vi "Error Check.vi"(8 "Error In":errorcluster, 9 "Next State Queue":refnum<queue>, 10 "Acquired Traces Queue":refnum<queue>) -> (0 "error out":errorcluster, 1 "Next State Queue":refnum<queue>, 2 "Acquired Traces Queue":refnum<queue>, 4 "Next State":T1, 5 "Error":bool)   [LabVIEW 2019]
uses:
  Controls/DAQ States.ctl
  Controls/Acquisition Result.ctl
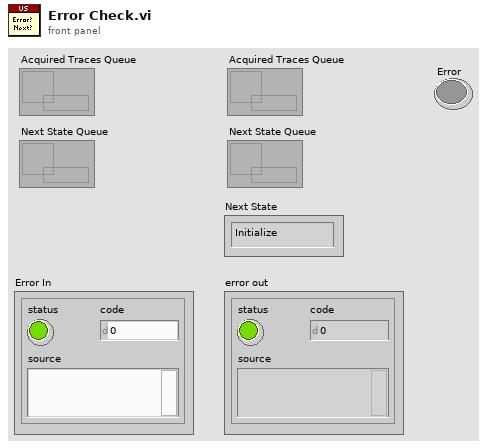
[diagram p1: front panel]
types:
  T1 = typedef "DAQ States.ctl" = enum16{"Initialize", "Idle", "Set Horizontal", "Set Vertical", "Set Trigger", "Set Display", "Acquire", "Analyze", "Set Switch", "Shutdown", "Quit"}
  T2 = typedef "Acquisition Result.ctl" = cluster{"Traces":waveform(sgl)[], "Relative t0 [s]":dbl, "Sample Rate [1/s]":dbl, "No. of points":i32, "Absolute t0 [s]":dbl, "dT [s]":dbl, "Update rate [1/s]":dbl, "Auto Triggered":bool, "Stop":bool}
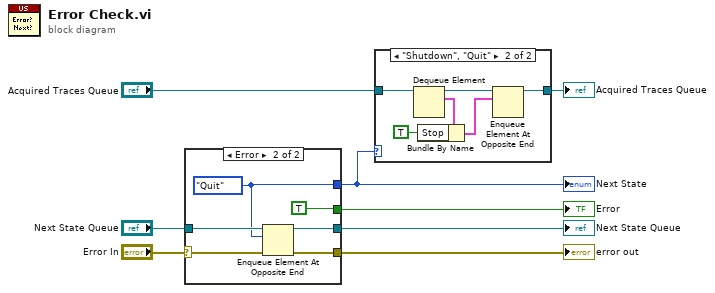
[diagram p0: block diagram]
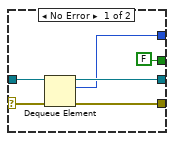
[diagram p3: hidden frame]
diagram:
  n1 = case shown="Error" "Error In" {
    selector: "Error In" -> [w10 w19]
    tunnel: "Next State Queue" -> [w14 w16]
    tunnel: [w13 w17] -> w8
    tunnel: [w12 w15] -> w1
    tunnel: [w11 w19] -> w6
    tunnel: [FALSE ("Error") TRUE ("Error")] -> w7
    frame No Error {
      n2 = Dequeue Element(queue=w14, error in (no error)=w10) -> (queue out=w13:refnum<queue>, element=w12:T1, error out=w11:errorcluster)  [unwired: 1 in, 1 out]
    }
    frame Error {
      w15 = DAQ_States."Quit" ("element")
      n3 = Enqueue Element At Opposite End(queue=w16, element=w15) -> (queue out=w17:refnum<queue>)  [unwired: 2 in, 2 out]
    }
  }
  "Next State Queue" <- w8
  "Next State" <- w1
  "Error" <- w7
  "error out" <- w6
  n4 = case shown="\"Shutdown\", \"Quit\"" w1 {
    tunnel: "Acquired Traces Queue" -> [w20 w26]
    tunnel: [w20 w21] -> w2
    frame "Initialize", Default {
    }
    frame "Shutdown", "Quit" {
      n5 = Dequeue Element(queue=w26) -> (queue out=w23:refnum<queue>, element=w24:T2)  [unwired: 2 in, 2 out]
      n6 = Bundle By Name(cluster=w24, "Stop"=TRUE) -> (w25:T2)
      n7 = Enqueue Element At Opposite End(queue=w23, element=w25) -> (queue out=w21:refnum<queue>)  [unwired: 2 in, 2 out]
    }
  }
  "Acquired Traces Queue" <- w2
